vi "Set Data.vi"(6 "Connector array":refnum<vi>[](array[refnum]), 9 "SlotNum":i32, 10 "Connector Type":T1, 11 "Data":T2 {"Input sources" items=["--unused--", "Probe Mic Right", "Probe Mic Left", "Cal Mic", "ABR", "CAP Right", "CAP Left", "Startle piezo", "Temperature", "Heart rate", "Accelerometer", "Startle piezo 2"]; "Output sources" items=["--unused--", "Right primary", "Right secondary", "Left primary", "Left secondary", "Shocks", "Startle", "Background", "Shaker", "Blue laser"]}) -> (2 "Connector Type out":T1, 3 "Data out":T2 {"Input sources" items=["--unused--", "Probe Mic Right", "Probe Mic Left", "Cal Mic", "ABR", "CAP Right", "CAP Left", "Startle piezo", "Temperature", "Heart rate", "Accelerometer", "Startle piezo 2"]; "Output sources" items=["--unused--", "Right primary", "Right secondary", "Left primary", "Left secondary", "Shocks", "Startle", "Background", "Shaker", "Blue laser"]})   [LabVIEW 2020, in "PXISlot.xctl"]
uses:
  PXISlot.xctl
  Data.ctl
  Output sources.ctl
  Input sources.ctl
  Connector Type.ctl
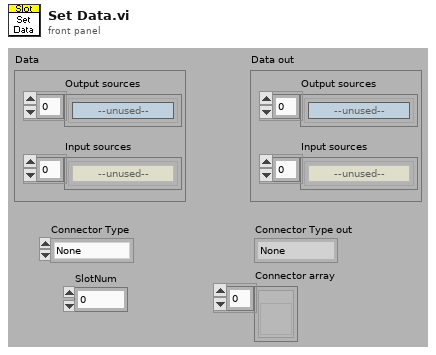
[diagram p1: front panel]
types:
  T1 = typedef "Connector Type.ctl" = enum16{"None", "PXI-4461", "BNC-2110", "BNC-2090", "PXIe-4463", "PXIe-4464"}
  T2 = typedef "PXISlot.xctl/Data.ctl" = cluster{"Output sources":T3[], "Input sources":T4[]}
  T3 = typedef "Output sources.ctl" = u16
  T4 = typedef "Input sources.ctl" = u16
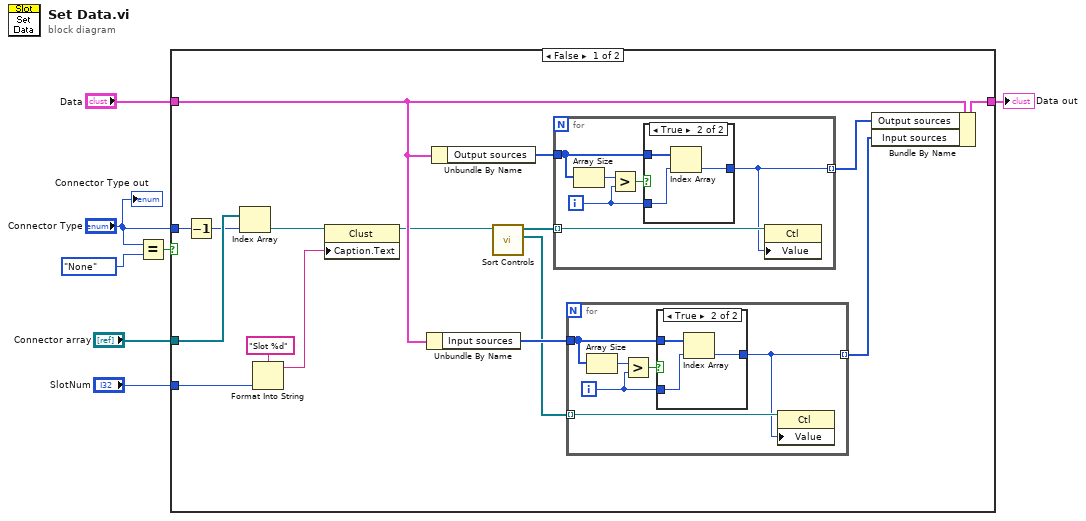
[diagram p0: block diagram]
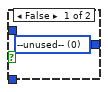
[diagram p2: hidden frame]
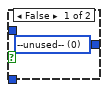
[diagram p3: hidden frame]
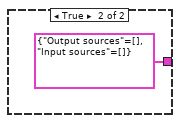
[diagram p4: hidden frame]
diagram:
  n1 = Equal?(x="Connector Type", y=Connector_Type."None") -> (x = y?=w5:bool)
  n2 = case shown="False" w5 {
    tunnel: "Data" -> [w21 _]
    tunnel: [w17 T2 {"Output sources"=[], "Input sources"=[]} ("Data")] -> w6
    tunnel: "Connector Type" -> [w14 _]
    tunnel: "Connector array" -> [w15 _]
    tunnel: "SlotNum" -> [w9 _]
    frame False {
      n3 = Decrement(x=w14) -> (x-1=w13:T1)
      n4 = Index Array(array=w15, index=w13) -> (element=w12:refnum<vi>)
      n5 = Format Into String(format string="Slot %d", w9) -> (resulting string=w8:string)  [unwired: 2 in, 1 out]
      n6 = property class="Clust"(reference=w12, "Caption.Text"=w8) -> (reference out=w11:refnum<vi>)  [unwired: 1 in, 1 out]
      n7 = Unbundle By Name(w21) -> ("Input sources"=w20:T4[])
      n8 = Unbundle By Name(w21) -> ("Output sources"=w23:T3[])
      n9 = call "Sort Controls.vi"("cluster ref"=w11) -> ("AI controls"=w16:refnum<vi>[], "AO controls"=w19:refnum<vi>[])  [unwired: 9 in]
      n10 = for {
        tunnel: w23 -> [w36]
        tunnel: w19 -> [w39] mode=indexing
        tunnel: [w34] -> w22 mode=indexing
        i -> [w35]
        n11 = Array Size(array=w36) -> (size(s)=w38:i32)
        n12 = Greater?(x=w38, y=w35) -> (0:w37:bool)
        n13 = case shown="True" w37 {
          tunnel: w36 -> [_ w43]
          tunnel: w35 -> [_ w42]
          tunnel: [w40 w41] -> w34
          frame False {
            w40 = T3 0 items=["--unused--", "Right primary", "Right secondary", "Left primary", "Left secondary", "Shocks", "Startle", "Background"] ("Ring")
          }
          frame True {
            n14 = Index Array(array=w43, index=w42) -> (element=w41:T3)
          }
        }
        n15 = property class="Ctl"(reference=w39, "Value"=w34) -> ()  [unwired: 1 in, 2 out]
      }
      n16 = for {
        tunnel: w20 -> [w26]
        tunnel: w16 -> [w29] mode=indexing
        tunnel: [w24] -> w18 mode=indexing
        i -> [w25]
        n17 = Array Size(array=w26) -> (size(s)=w28:i32)
        n18 = Greater?(x=w28, y=w25) -> (0:w27:bool)
        n19 = case shown="True" w27 {
          tunnel: w26 -> [_ w33]
          tunnel: w25 -> [_ w32]
          tunnel: [w30 w31] -> w24
          frame False {
            w30 = T3 0 items=["--unused--", "Right primary", "Right secondary", "Left primary", "Left secondary", "Shocks", "Startle", "Background"] ("Ring")
          }
          frame True {
            n20 = Index Array(array=w33, index=w32) -> (element=w31:T4)
          }
        }
        n21 = property class="Ctl"(reference=w29, "Value"=w24) -> ()  [unwired: 1 in, 2 out]
      }
      n22 = Bundle By Name(cluster=w21, "Output sources"=w22, "Input sources"=w18) -> (w17:T2)
    }
    frame True {
    }
  }
  "Data out" <- w6
  "Connector Type out" <- "Connector Type"
